vi "Open-Graph.vi"() -> ()   [LabVIEW 2014]
uses:
  <vilib>/Utility/file.llb/Read From Spreadsheet File (DBL).vi
panel:
  out "XY Graph":cluster{dbl[], dbl[]}(graph)
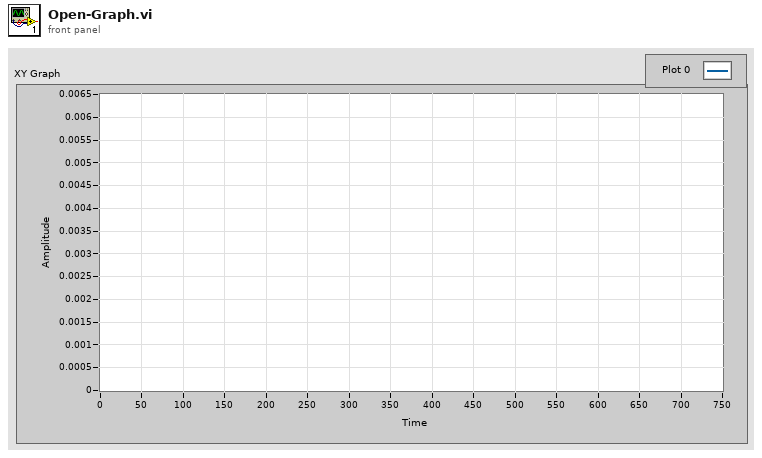
[diagram p1: front panel]
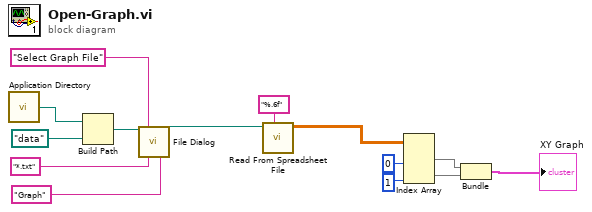
[diagram p0: block diagram]
diagram:
  n1 = call <vilib>:"Application Directory.vi"() -> ("Application Directory"=w9:path)
  n2 = Build Path(base path=w9, name or relative path=path "data") -> (appended path=w8:path)
  n3 = call "File Dialog"("start path"=w8, "prompt"="Select Graph File", "pattern (all files)"="*.txt", "pattern label"="Graph") -> ("selected path"=w11:path)  [unwired: 8 in, 3 out]
  n4 = call-poly <vilib>:"Read From Spreadsheet File.vi"("format (%.3f)"="%.6f", "file path (dialog if empty)"=w11) -> ("all rows"=w1:dbl[][])  [unwired: 5 in, 4 out]
  n5 = Index Array(array=w1, index (col) #1=0 ("index (row)"), index (col) #2=1 ("index (row)")) -> (element #1=w6:dbl[], element #2=w5:dbl[])  [unwired: 2 in]
  n6 = Bundle("all rows"=w6, "all rows"=w5) -> (→"XY Graph":cluster{"all rows":dbl[], "all rows":dbl[]})  [unwired: 1 in]
